vi "open.vi"(8 "error in (no error)":errorcluster, 11 "SerialConnection in":refnum<class "SerialConnection.lvclass">) -> (0 "error out":errorcluster, 3 "SerialConnection out":refnum<class "SerialConnection.lvclass">)   [LabVIEW 2023, in "SerialConnection.lvclass"]
uses:
  SerialConnection.lvclass
  SerialConnection.lvclass/SerialConnection.ctl
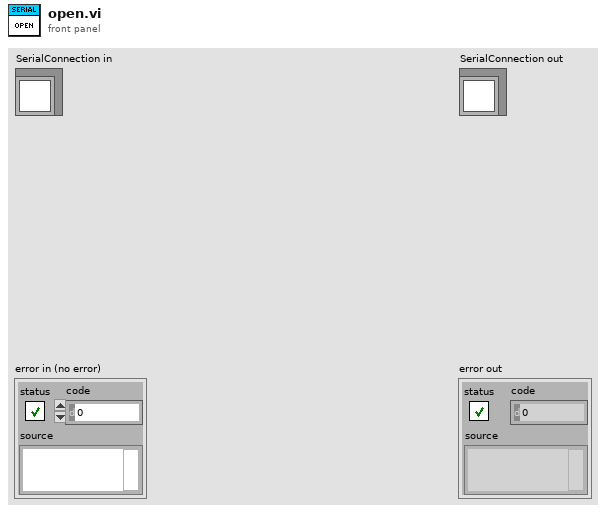
[diagram p1: front panel]
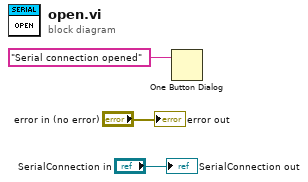
[diagram p0: block diagram]
diagram:
  n1 = One Button Dialog(message="Serial connection opened") -> ()  [unwired: 1 in, 1 out]
  "error out" <- "error in (no error)"
  "SerialConnection out" <- "SerialConnection in"
